vi "write_attributes.vi"(8 "error in (no error)":errorcluster, 10 "attributes":T1, 11 "NMF in":refnum<class "NMF.lvclass">) -> (0 "error out":errorcluster, 3 "NMF out":refnum<class "NMF.lvclass">)   [LabVIEW 2020, in "NMF.lvclass"]
uses:
  NMF.lvclass
  Controls/non_negative_matrix_factorization_attributes.ctl
  NMF.lvclass/NMF.ctl
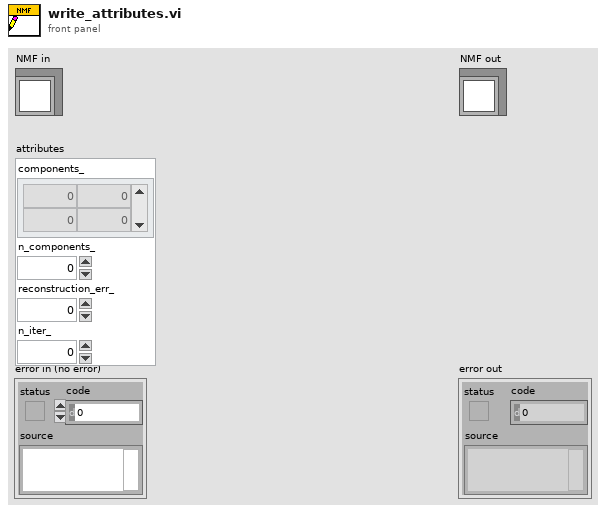
[diagram p1: front panel]
types:
  T1 = typedef "non_negative_matrix_factorization_attributes.ctl" = cluster{"components_":dbl[][], "n_components_":dbl, "reconstruction_err_":dbl, "n_iter_":dbl}
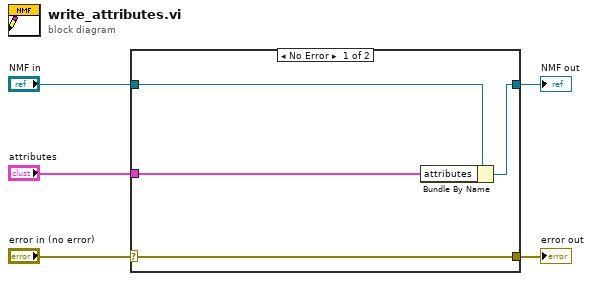
[diagram p0: block diagram]
diagram:
  n1 = case shown="No Error" "error in (no error)" {
    selector: "error in (no error)" -> [w9 w10]
    tunnel: [w9 w10] -> w4
    tunnel: [w7 w11] -> w2
    tunnel: "NMF in" -> [w8 w11]
    tunnel: "attributes" -> [w6 _]
    frame No Error {
      n2 = Bundle By Name(cluster=w8, "attributes"=w6) -> (w7:refnum<class "NMF.lvclass">)
    }
    frame Error {
    }
  }
  "error out" <- w4
  "NMF out" <- w2
